vi "Microstrain Test.vi"() -> ()   [LabVIEW 2011]
uses:
  <instrlib>/MicroStrain 3DM-GX1/MicroStrain 3DM-GX1.lvlib
panel:
  out "Instrument Firmware Revision":string
  in  "stop":bool
  out "error out":errorcluster
  in  "Baud Rate (38400)":u32(ring)=115200 items=["19200"=19200, "38400"=38400, "115200"=115200]
  in  "VISA resource name":refnum<visa-resource-name>
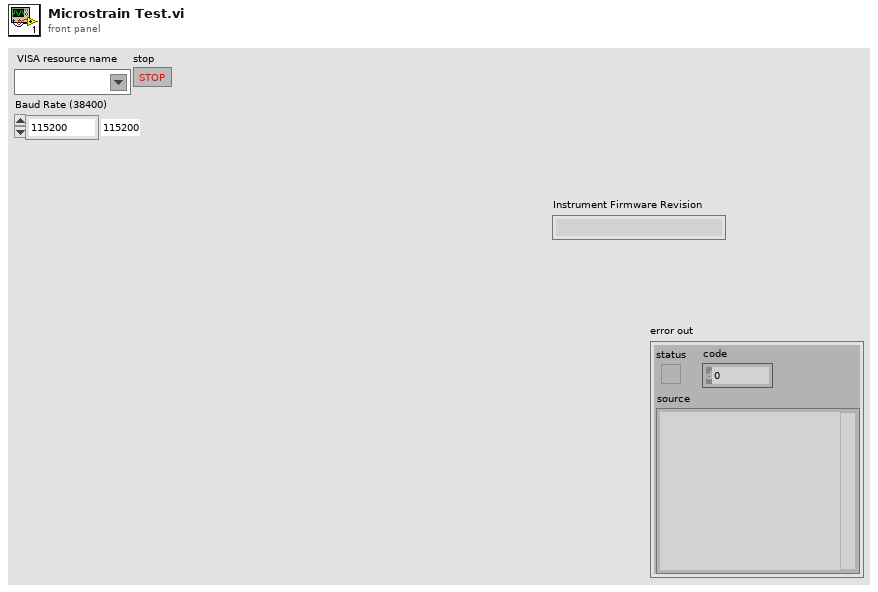
[diagram p1: front panel]
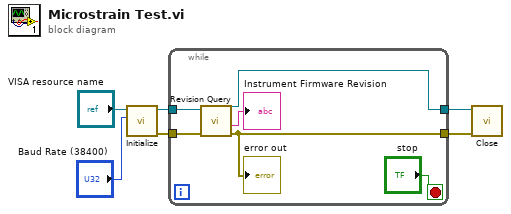
[diagram p0: block diagram]
diagram:
  n1 = call <instrlib>:"Initialize.vi"("Baud Rate (38400)"="Baud Rate (38400)", "VISA resource name"="VISA resource name") -> ("error out"=w3:errorcluster, "VISA resource name out"=w4:refnum<visa-resource-name>)  [unwired: 8 in]
  n2 = while {
    tunnel: w4 -> [w12]
    tunnel: w3 -> [w9]
    tunnel: [w11] -> w2
    tunnel: [w10] -> w1
    stop <- "stop" stop-if-true
    n3 = call <instrlib>:"Revision Query.vi"("error in (no error)"=w9, "VISA resource name"=w12) -> ("error out"=w10:errorcluster, "Instrument Firmware Revision"=→"Instrument Firmware Revision":string, "VISA resource name out"=w11:refnum<visa-resource-name>)  [unwired: 5 in, 2 out]
    "error out" <- w10
  }
  n4 = call <instrlib>:"Close.vi"("error in (no error)"=w1, "VISA resource name"=w2) -> ()  [unwired: 9 in, 1 out]
